vi "Is1DArray.vi"(3 "Datatype":T1, 4 "Value String in":string) -> (0 "IsArray":bool, 2 "Array Value":variant)   [LabVIEW 2016]
uses:
  Datatype.ctl
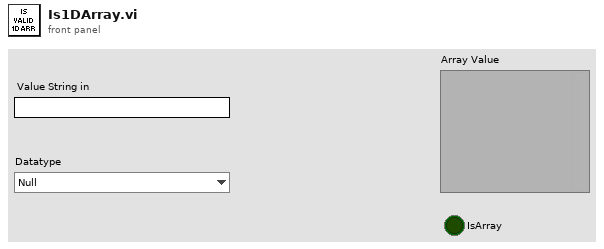
[diagram p1: front panel]
types:
  T1 = typedef "Datatype.ctl" = enum16{"Null", "Numeric", "String", "Bool", "Numeric 1D", "String 1D", "Bool 1D", "Numeric 2D", "String 2D", "Bool 2D", "Variant"}
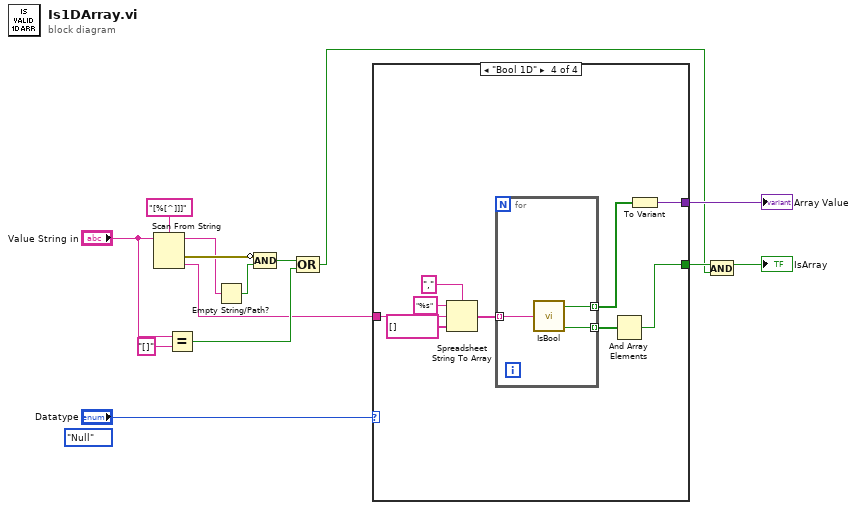
[diagram p0: block diagram]
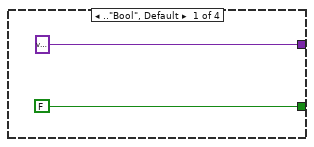
[diagram p2: hidden frame]
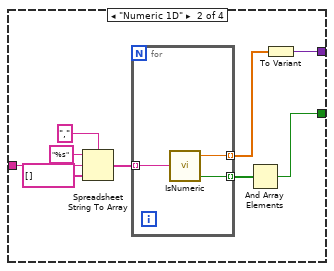
[diagram p3: hidden frame]
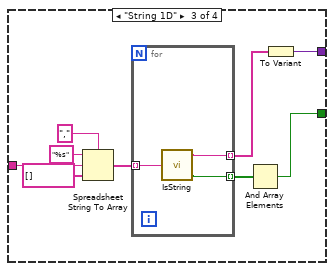
[diagram p4: hidden frame]
diagram:
  (unwired) Datatype."Null" ("Datatype")
  n1 = Scan From String(format string="[%[^]]]", input string="Value String in") -> (remaining string=w12:string, error out=w13:errorcluster, output 1=w3:string)  [unwired: 3 in, 1 out]
  n2 = Equal?(x="Value String in", y="[]") -> (x = y?=w7:bool)
  n3 = Empty String/Path?(string/path=w12) -> (empty?=w11:bool)
  n4 = Compound Arithmetic op=AND(invert w13, w11) -> (w10:bool)
  n5 = Compound Arithmetic op=OR(w10, w7) -> (w1:bool)
  n6 = case shown="\"Bool 1D\"" "Datatype" {
    tunnel: [FALSE w19 w31 w43] -> w5
    tunnel: [variant w18 w30 w42] -> w4
    tunnel: w3 -> [_ w23 w35 w47]
    frame .."Bool", Default {
    }
    frame "Numeric 1D" {
      n7 = Spreadsheet String To Array(delimiter (Tab)=",", format string="%s", spreadsheet string=w23, array type (2D Dbl)=string[] []) -> (array=w21:string[])
      n8 = for {
        tunnel: w21 -> [w28] mode=indexing
        tunnel: [w27] -> w17 mode=indexing
        tunnel: [w26] -> w20 mode=indexing
        n9 = call "IsNumeric.vi"("Value String in"=w28) -> ("IsNumeric"=w26:bool, "Numeric Value"=w27:ext)  [unwired: 3 in]
      }
      n10 = And Array Elements(Boolean array=w20) -> (logical AND=w19:bool)
      n11 = To Variant(anything=w17) -> (Variant=w18:variant)
    }
    frame "String 1D" {
      n12 = Spreadsheet String To Array(delimiter (Tab)=",", format string="%s", spreadsheet string=w35, array type (2D Dbl)=string[] []) -> (array=w33:string[])
      n13 = for {
        tunnel: w33 -> [w40] mode=indexing
        tunnel: [w39] -> w29 mode=indexing
        tunnel: [w38] -> w32 mode=indexing
        n14 = call "IsString.vi"("Value String in"=w40) -> ("IsString"=w38:bool, "String Value"=w39:string)  [unwired: 3 in]
      }
      n15 = And Array Elements(Boolean array=w32) -> (logical AND=w31:bool)
      n16 = To Variant(anything=w29) -> (Variant=w30:variant)
    }
    frame "Bool 1D" {
      n17 = Spreadsheet String To Array(delimiter (Tab)=",", format string="%s", spreadsheet string=w47, array type (2D Dbl)=string[] []) -> (array=w45:string[])
      n18 = for {
        tunnel: w45 -> [w52] mode=indexing
        tunnel: [w51] -> w41 mode=indexing
        tunnel: [w50] -> w44 mode=indexing
        n19 = call "IsBool.vi"("Value String in"=w52) -> ("IsBool"=w50:bool, "Bool Value"=w51:bool)  [unwired: 3 in]
      }
      n20 = And Array Elements(Boolean array=w44) -> (logical AND=w43:bool)
      n21 = To Variant(anything=w41) -> (Variant=w42:variant)
    }
  }
  "Array Value" <- w4
  n22 = And(x=w5, y=w1) -> (x .and. y?=→"IsArray":bool)
